vi "SW_Fire_TTL_during_the_acquisition.vi"(8 "error in (no error)":errorcluster, 9 "Serial Port In":refnum<visa-resource-name>="COM3", 10 "TTL port to fire":u8, 11 "Fire TTL":bool) -> (0 "error out":errorcluster)   [LabVIEW 2018]
doc: "Fires TTL High to the TTL2 output for ~250 ms (default)."
panel:
  out "TTL has been reset":bool=TRUE
  out "TTL is fired":bool
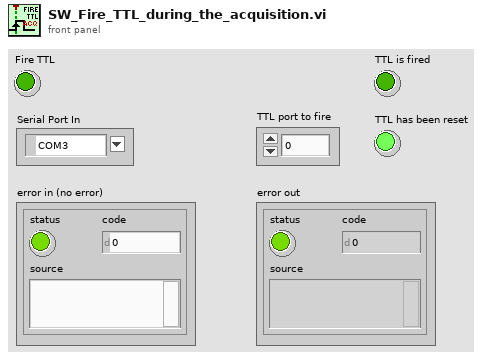
[diagram p1: front panel]
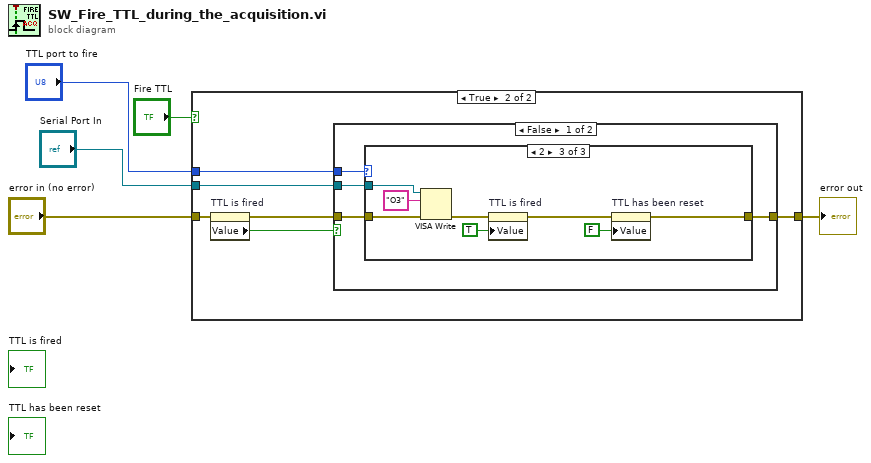
[diagram p0: block diagram]
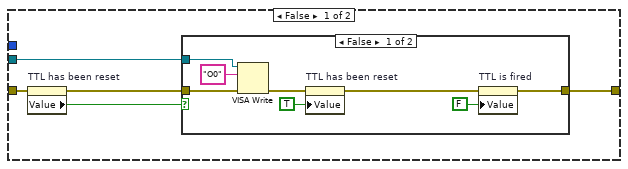
[diagram p2: hidden frame]
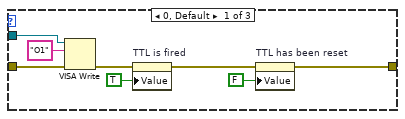
[diagram p4: hidden frame]
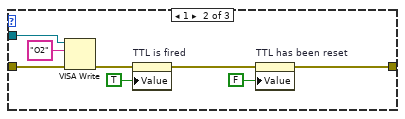
[diagram p5: hidden frame]
diagram:
  n1 = case shown="True" "Fire TTL" {
    tunnel: "TTL port to fire" -> [_ w23]
    tunnel: "Serial Port In" -> [w10 w25]
    tunnel: "error in (no error)" -> [w9 w22]
    tunnel: [w7 w24] -> w2
    frame False {
      n2 = property on="TTL has been reset" class="Bool (strict)"(error in=w9) -> (error out=w8:errorcluster, "Value"=w6:bool)  [unwired: 1 in, 1 out]
      n3 = case shown="False" w6 {
        tunnel: w8 -> [w17 w19]
        tunnel: [w11 w19] -> w7
        tunnel: w10 -> [w16 _]
        frame False {
          n4 = VISA Write(VISA resource name=w16, write buffer="O0" ("string"), error in (no error)=w17) -> (error out=w15:errorcluster)  [unwired: 2 out]
          n5 = property on="TTL has been reset" class="Bool (strict)"(error in=w15, "Value"=TRUE ("TTL has been reset")) -> (error out=w12:errorcluster)  [unwired: 1 in, 1 out]
          n6 = property on="TTL is fired" class="Bool (strict)"(error in=w12, "Value"=FALSE ("TTL is fired")) -> (error out=w11:errorcluster)  [unwired: 1 in, 1 out]
        }
        frame True {
        }
      }
    }
    frame True {
      n7 = property on="TTL is fired" class="Bool (strict)"(error in=w22) -> (error out=w21:errorcluster, "Value"=w20:bool)  [unwired: 1 in, 1 out]
      n8 = case shown="False" w20 {
        tunnel: w25 -> [w29 _]
        tunnel: w21 -> [w28 w54]
        tunnel: [w27 w54] -> w24
        tunnel: w23 -> [w26 _]
        frame False {
          n9 = case shown="2" w26 {
            tunnel: w29 -> [w36 w44 w52]
            tunnel: w28 -> [w35 w43 w51]
            tunnel: [w31 w39 w47] -> w27
            frame 0, Default {
              n10 = VISA Write(VISA resource name=w36, write buffer="O1" ("string"), error in (no error)=w35) -> (error out=w33:errorcluster)  [unwired: 2 out]
              n11 = property on="TTL is fired" class="Bool (strict)"(error in=w33, "Value"=TRUE ("TTL is fired")) -> (error out=w32:errorcluster)  [unwired: 1 in, 1 out]
              n12 = property on="TTL has been reset" class="Bool (strict)"(error in=w32, "Value"=FALSE ("TTL has been reset")) -> (error out=w31:errorcluster)  [unwired: 1 in, 1 out]
            }
            frame 1 {
              n13 = VISA Write(VISA resource name=w44, write buffer="O2" ("string"), error in (no error)=w43) -> (error out=w41:errorcluster)  [unwired: 2 out]
              n14 = property on="TTL is fired" class="Bool (strict)"(error in=w41, "Value"=TRUE ("TTL is fired")) -> (error out=w40:errorcluster)  [unwired: 1 in, 1 out]
              n15 = property on="TTL has been reset" class="Bool (strict)"(error in=w40, "Value"=FALSE ("TTL has been reset")) -> (error out=w39:errorcluster)  [unwired: 1 in, 1 out]
            }
            frame 2 {
              n16 = VISA Write(VISA resource name=w52, write buffer="O3" ("string"), error in (no error)=w51) -> (error out=w49:errorcluster)  [unwired: 2 out]
              n17 = property on="TTL is fired" class="Bool (strict)"(error in=w49, "Value"=TRUE ("TTL is fired")) -> (error out=w48:errorcluster)  [unwired: 1 in, 1 out]
              n18 = property on="TTL has been reset" class="Bool (strict)"(error in=w48, "Value"=FALSE ("TTL has been reset")) -> (error out=w47:errorcluster)  [unwired: 1 in, 1 out]
            }
          }
        }
        frame True {
        }
      }
    }
  }
  "error out" <- w2
